vi "find index of the image name.vi"(8 "error in (no error)":errorcluster, 11 "Channel in":refnum<class "SPARC4_Channel.lvclass">) -> (0 "error out":errorcluster, 3 "Channel out":refnum<class "SPARC4_Channel.lvclass">)   [LabVIEW 2018, in "SPARC4_Channel.lvclass"]
doc: "Find the index of the lastest image in the current directory"
uses:
  SPARC4_Channel.lvclass
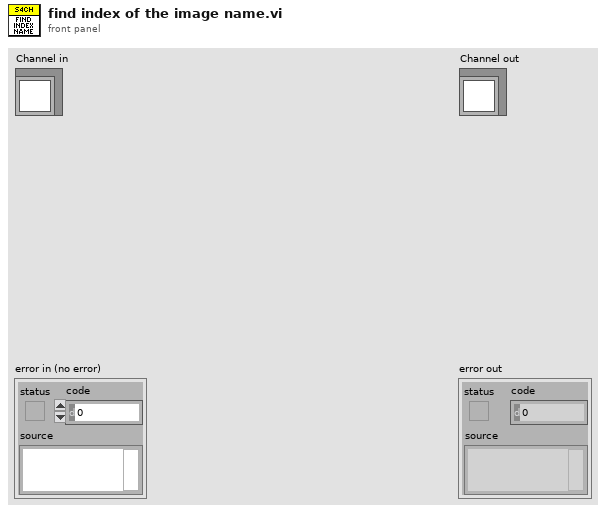
[diagram p1: front panel]
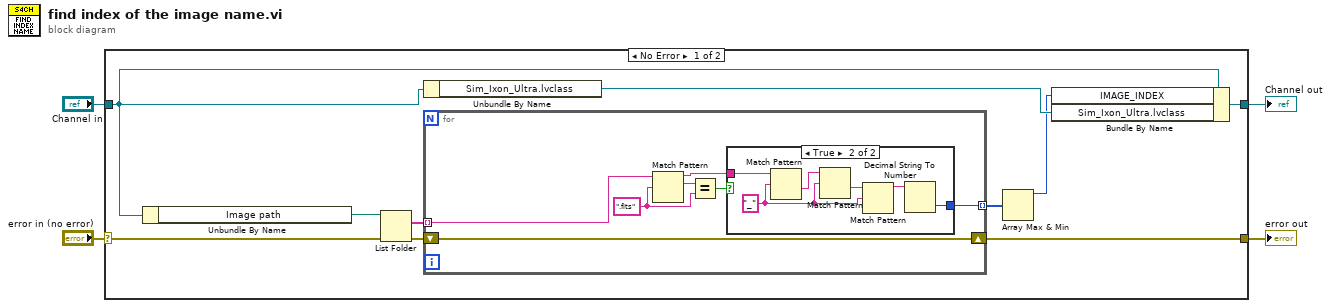
[diagram p0: block diagram]
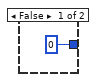
[diagram p2: hidden frame]
diagram:
  n1 = case shown="No Error" "error in (no error)" {
    selector: "error in (no error)" -> [w14 w30]
    tunnel: [w8 w30] -> w3
    tunnel: [w11 w29] -> w1
    tunnel: "Channel in" -> [w10 w29]
    frame No Error {
      n2 = Unbundle By Name(w10) -> ("Image path"=w6:path)
      n3 = List Folder(path=w6, error in=w14) -> (filenames=w12:string[], error out=w13:errorcluster)  [unwired: 2 in, 2 out]
      n4 = Unbundle By Name(w10) -> ("Sim_Ixon_Ultra.lvclass"=w9:refnum<class "Sim_Ixon_Ultra.lvclass">)
      n5 = for {
        shift-right: [w21] -> w8
        shift-left: w13 -> [w21]
        tunnel: w12 -> [w18] mode=indexing
        tunnel: [w19] -> w7 mode=indexing
        w16 = ".fits" ("regular expression")
        n6 = Match Pattern(string=w18, regular expression=w16) -> (before substring=w20:string, match substring=w17:string)  [unwired: 1 in, 2 out]
        n7 = Equal?(x=w17, y=w16) -> (x = y?=w15:bool)
        n8 = case shown="True" w15 {
          tunnel: w20 -> [_ w27]
          tunnel: [0 w28] -> w19
          frame False {
          }
          frame True {
            w24 = "_" ("regular expression")
            n9 = Match Pattern(string=w27, regular expression=w24) -> (after substring=w26:string)  [unwired: 1 in, 3 out]
            n10 = Match Pattern(string=w26, regular expression=w24) -> (after substring=w25:string)  [unwired: 1 in, 3 out]
            n11 = Match Pattern(string=w25, regular expression=w24) -> (before substring=w23:string)  [unwired: 1 in, 3 out]
            n12 = Decimal String To Number(string=w23) -> (number=w28:i32)  [unwired: 2 in, 1 out]
          }
        }
      }
      n13 = Array Max & Min(array=w7) -> (max value=w5:i32)  [unwired: 3 out]
      n14 = Bundle By Name(cluster=w10, "IMAGE_INDEX"=w5, "Sim_Ixon_Ultra.lvclass"=w9) -> (w11:refnum<class "SPARC4_Channel.lvclass">)
    }
    frame Error {
    }
  }
  "error out" <- w3
  "Channel out" <- w1
